vi "DefaultFromINI.vi"(8 "error in (no error)":errorcluster, 11 "PacificPowerSource":refnum<class "PacificPowerSource.lvclass">) -> (0 "error out":errorcluster, 3 "PacificPowerSource":refnum<class "PacificPowerSource.lvclass">)   [LabVIEW 2018, in "AcPwrPlugins.lvlib" / "PacificPowerSource.lvclass"]
doc: "This VI reads the properties from the INI file and puts them into the LabVIEW class for further use."
uses:
  PacificPowerSource.lvclass
  C:/Program Files (x86)/National Instruments/LabVIEW 2018/user.lib/NIST/BaseClasses/BasePlugin_class/BasePlugin.lvclass
  C:/Users/Public/Projects/ICDAS/NistPluggableModules/AcPwr/AcPwrPlugins/AcPwrBaseClass/AcPwrBase.lvclass
  TypeDefs/Device(s)Settings.ctl
  TypeDefs/Measurements.ctl
  TypeDefs/MeasurementType.ctl
  <userlib>/NIST/BaseClasses/BasePlugin_class/BasePlugin.lvclass/BasePlugin.ctl
  <userlib>/NIST/BaseClasses/BasePlugin_class/Accessors/Read PluginIniFilePath.vi
  AcPwrBaseClass/AcPwrBase.lvclass
  <vilib>/Utility/config.llb/NI_LVConfig.lvlib
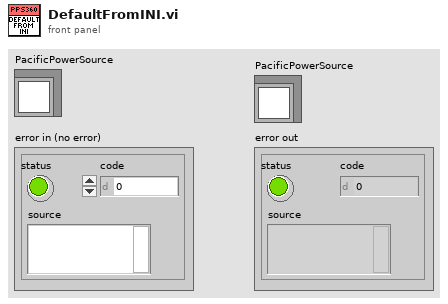
[diagram p1: front panel]
types:
  T1 = typedef "AcPwrPlugins.lvlib/PacificPowerSource.lvclass/Measurements.ctl" = cluster{"Handle":string, "Name":string, "Enabled ":bool, "Measurement Value":dbl, "Channel Name":enum16{"A", "B", "C"}, "Measurement Type ":T2}[]
  T2 = typedef "AcPwrPlugins.lvlib/PacificPowerSource.lvclass/MeasurementType.ctl" = enum16{"Voltage RMS L-N", "Voltage RMS L-L", "Frequency", "Current RMS", "Current Peak", "Crest Factor", "Power Factor", "Power VA", "Real Power"}
  T3 = typedef "AcPwrPlugins.lvlib/PacificPowerSource.lvclass/Device(s)Settings.ctl" = cluster{"MeasName":string, "Modules":cluster{"Handle":string, "Connected":bool, "Clear Device (F)":bool, "btnIdQuery":bool, "btnReset":bool, "Program #":cluster{"Phase B (Degrees)":i32, "Waveform A (1: Sine)":i32, "Voltage Level (Va)":dbl, "Program Number (0)":i32, "Voltage Level (Vb) ":dbl, "Form (3: Three)":u16, "Coupling  (0: Direct)":u16, "Frequency (45Hz)":dbl, "Current Limit (40A)":dbl, "Phase C (Degrees)":i32, "Voltage Level (Vc)":dbl, "Waveform B (1: Sine)":i32, "Waveform C (1: Sine)":i32}[], "Impedance Parameters (off, 0.00)":cluster{"State":bool, "Impedance":dbl}, "Transient Execution (F)":bool, "OutputEnabled":bool, "Source Range":cluster{"Frequency Minimum (45 Hz)":dbl, "Frequency Maximum (1200 Hz)":dbl, "Voltage Maximum (V)":dbl, "Voltage Minimum (V)":dbl, "Range Control (0: Auto)":u16, "Initial Voltage (0V)":u16, "Frequency Range (600Hz)":u16}, "Port Type":enum16{"GPIB", "Serial"}}[]}
  T4 = typedef "NI_LVConfig.lvlib/Config Data RefNum.ctl" = refnum<k1>
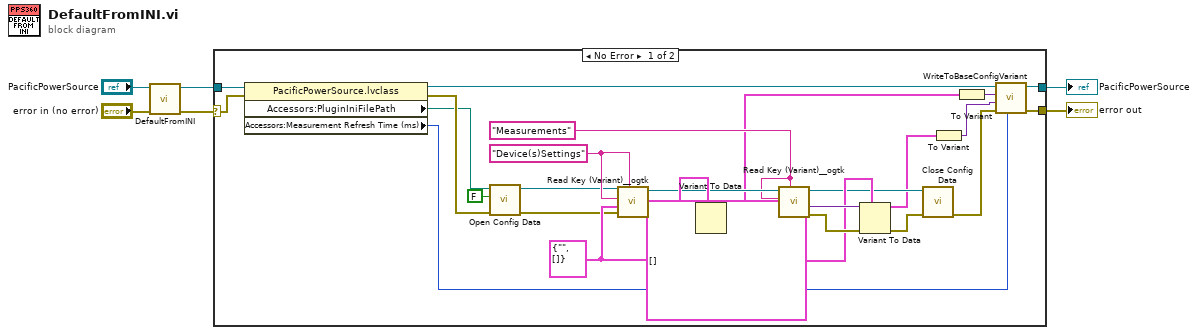
[diagram p0: block diagram]
diagram:
  n1 = call-parent "DefaultFromINI.vi"("error in (no error)"="error in (no error)", "AcPwrBase"="PacificPowerSource") -> ("error out"=w1:errorcluster, "AcPwrBase"=w2:refnum<class "PacificPowerSource.lvclass">)  [unwired: 8 in]
  n2 = case shown="No Error" w1 {
    selector: w1 -> [w33 w35]
    tunnel: [w11 w35] -> w6
    tunnel: [w12 w36] -> w5
    tunnel: w2 -> [w34 w36]
    frame No Error {
      w22 = "Measurements" ("section")
      w21 = T1 [] ("Measurements")
      w24 = T3 {"MeasName"="", "Modules"=[]} ("Load Settings")
      w25 = "Device(s)Settings" ("section")
      n3 = property class="PacificPowerSource.lvclass"(reference=w34, error in=w33) -> (reference out=w14:refnum<class "PacificPowerSource.lvclass">, error out=w32:errorcluster, "Accessors:PluginIniFilePath"=w31:path, "Accessors:Measurement Refresh Time (ms)"=w9:u32)
      n4 = call <vilib>:"Open Config Data.vi"("error in (no error)"=w32, "create file if necessary (T)"=FALSE, "configuration file path"=w31) -> ("error out"=w18:errorcluster, "refnum"=w17:T4)  [unwired: 6 in, 1 out]
      n5 = call <userlib>:"Read Key (Variant)__ogtk.vi"("section"=w25, "error in (no error)"=w18, "type"=w24, "key (optional)"=w25, "refnum"=w17) -> ("error out"=w29:errorcluster, "key-value"=w30:variant, "refnum out"=w23:T4)  [unwired: 3 in, 1 out]
      n6 = Variant To Data(error in=w29, type=w24, Variant=w30) -> (data=w13:T3, error out=w26:errorcluster)
      n7 = call <userlib>:"Read Key (Variant)__ogtk.vi"("section"=w22, "error in (no error)"=w26, "type"=w21, "key (optional)"=w22, "refnum"=w23) -> ("error out"=w28:errorcluster, "key-value"=w27:variant, "refnum out"=w19:T4)  [unwired: 3 in, 1 out]
      n8 = Variant To Data(error in=w28, type=w21, Variant=w27) -> (data=w8:T1, error out=w20:errorcluster)
      n9 = call <vilib>:"Close Config Data.vi"("error in (no error)"=w20, "refnum"=w19) -> ("error out"=w15:errorcluster)  [unwired: 8 in, 1 out]
      n10 = To Variant(anything=w8) -> (Variant=w7:variant)
      n11 = To Variant(anything=w13) -> (Variant=w16:variant)
      n12 = call "WriteToBaseConfigVariant.vi"("Measurement Refresh Time (ms)"=w9, "error in (no error)"=w15, "Meas"=w7, "Config"=w16, "PacificPowerSource in"=w14) -> ("error out"=w11:errorcluster, "PacificPowerSource out"=w12:refnum<class "PacificPowerSource.lvclass">)  [unwired: 5 in]
    }
    frame Error {
    }
  }
  "error out" <- w6
  "PacificPowerSource" <- w5
